vi "get_scan_status.vi"(8 "error in":errorcluster, 11 "address":string) -> (0 "Scanning Blue?":bool, 1 "Scanning Red?":bool, 2 "Reducing Errors?":bool, 3 "Scan Finished?":bool, 4 "error out":errorcluster)   [LabVIEW 2020]
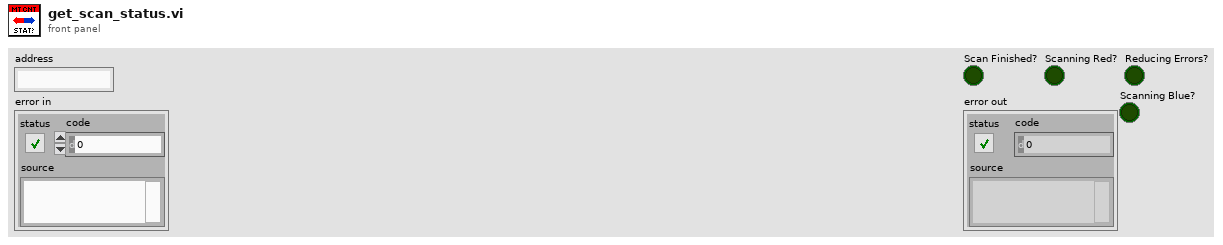
[diagram p1: front panel]
types:
  T1 = enum16{"Standard", "Buffered", "CRLF", "Immediate"}
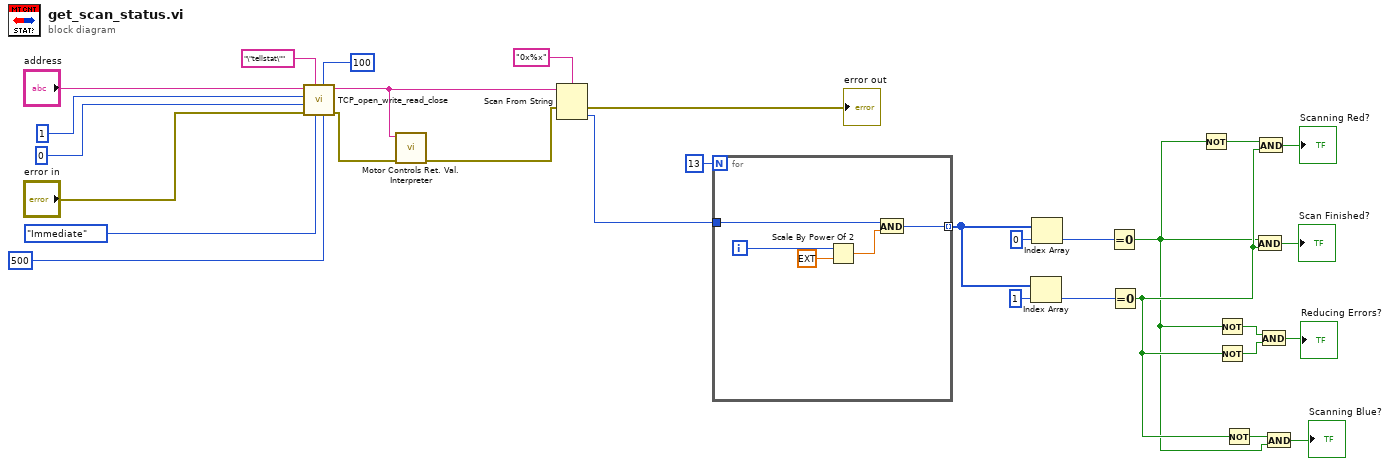
[diagram p0: block diagram]
diagram:
  n1 = call "TCP_open_write_read_close.vi"("timeout ms (25000)"=500, "bytes to read"=100, "mode (standard)"=T1."Immediate", "write string"="\"tellstat\"", "error in"="error in", "local port (0)"=u16 0, "remote port or service name"=u16 1, "address"="address") -> ("error out"=w24:errorcluster, "read string"=w22:string)  [unwired: 2 in]
  n2 = call "Motor Controls Ret. Val. Interpreter.vi"("error in"=w24, "Command Return"=w22) -> ("error out"=w20:errorcluster)  [unwired: 8 in, 1 out]
  n3 = Scan From String(format string="0x%x", input string=w22, error in=w20) -> (error out=→"error out":errorcluster, output 1=w18:u32)  [unwired: 2 in, 2 out]
  n4 = for {
    N: 13 -> [_]
    tunnel: w18 -> [w35]
    tunnel: [w31] -> w16 mode=indexing
    i -> [w33]
    n5 = Scale By Power Of 2(n=w33, x=ext 1.0) -> (x*2^n=w34:ext)
    n6 = And(x=w35, y=w34) -> (x .and. y?=w31:i32)
  }
  n7 = Index Array(array=w16, index=1) -> (element=w12:i32)
  n8 = Index Array(array=w16, index=0) -> (element=w13:i32)
  n9 = Equal To 0?(x=w13) -> (x = 0?=w2:bool)
  n10 = Equal To 0?(x=w12) -> (x = 0?=w3:bool)
  n11 = Not(x=w2) -> (.not. x?=w9:bool)
  n12 = Not(x=w2) -> (.not. x?=w8:bool)
  n13 = Not(x=w3) -> (.not. x?=w7:bool)
  n14 = Not(x=w3) -> (.not. x?=w4:bool)
  n15 = And(x=w2, y=w3) -> (x .and. y?=→"Scan Finished?":bool)
  n16 = And(x=w9, y=w3) -> (x .and. y?=→"Scanning Red?":bool)
  n17 = And(x=w8, y=w7) -> (x .and. y?=→"Reducing Errors?":bool)
  n18 = And(x=w4, y=w2) -> (x .and. y?=→"Scanning Blue?":bool)
